vi "Execution Hierarchy.vi"() -> (2 "Top Level VI Name":string)   [LabVIEW 2022 SP3, in "FlexBlocks Support.lvlib"]
uses:
  FlexBlocks Support.lvlib
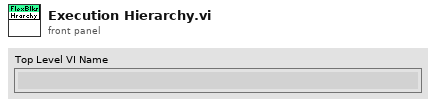
[diagram p1: front panel]
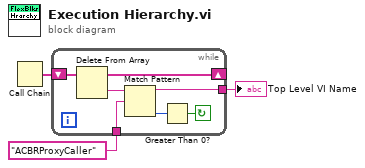
[diagram p0: block diagram]
diagram:
  n1 = Call Chain() -> (call chain=w3:string[])
  n2 = while {
    tunnel: [w6] -> w1
    shift-right: [w7] -> _
    shift-left: w3 -> [w10]
    tunnel: "ACBRProxyCaller" -> [w8]
    stop <- w4 continue-if-true
    n3 = Delete From Array(array=w10) -> (deleted portion=w9:string, array with subset deleted=w7:string[])  [unwired: 2 in]
    n4 = Match Pattern(string=w9, regular expression=w8) -> (before substring=w6:string, offset past match=w5:i32)  [unwired: 1 in, 2 out]
    n5 = Greater Than 0?(x=w5) -> (x > 0?=w4:bool)
  }
  "Top Level VI Name" <- w1
